vi "Check Workflow.vi"(9 "Part In":map{string, i64}(c390), 10 "Current  Workflow":string, 11 "Workflow Map":map{string, string[]}(c390)) -> (3 "Accepted?":bool)   [LabVIEW 2021]
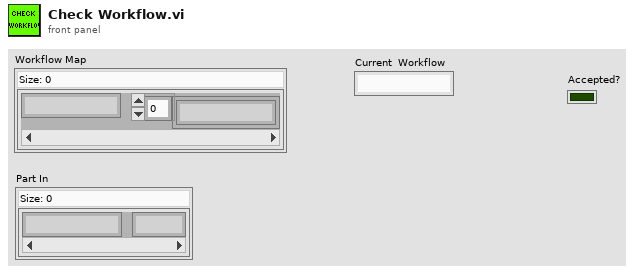
[diagram p1: front panel]
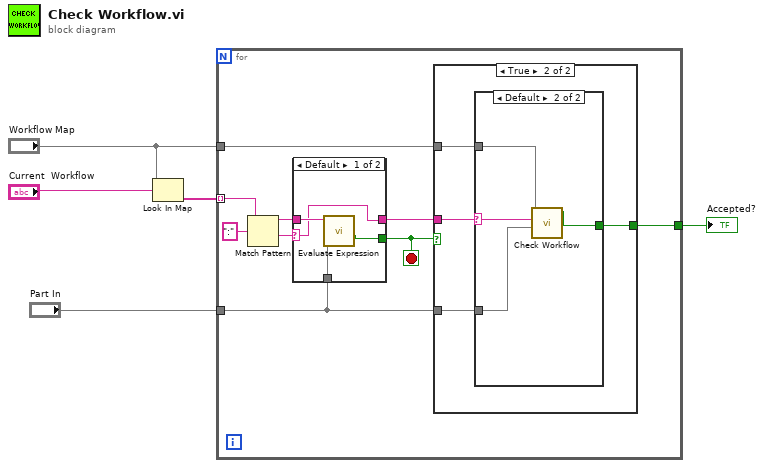
[diagram p0: block diagram]
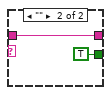
[diagram p2: hidden frame]
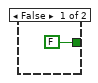
[diagram p3: hidden frame]
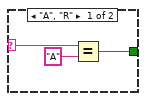
[diagram p4: hidden frame]
diagram:
  n1 = Look In Map(map="Workflow Map", key="Current  Workflow") -> (value=w4:string[])  [unwired: 1 in, 1 out]
  n2 = for {
    tunnel: w4 -> [w14] mode=indexing
    tunnel: "Workflow Map" -> [w8]
    tunnel: "Part In" -> [w6]
    tunnel: [w7] -> w1
    stop <- w9 stop-if-true
    n3 = Match Pattern(string=w14, regular expression=":") -> (before substring=w11:string, after substring=w12:string)  [unwired: 1 in, 2 out]
    n4 = case shown="Default" w12 {
      selector: w12 -> [w15 _]
      tunnel: [w16 TRUE] -> w9
      tunnel: w11 -> [w18 w19]
      tunnel: [w15 w19] -> w10
      tunnel: w6 -> [w17 _]
      frame Default {
        n5 = call "Evaluate Expression.vi"("Part In"=w17, "Expression"=w18) -> ("Pass/Fail"=w16:bool)  [unwired: 9 in]
      }
      frame "" {
      }
    }
    n6 = case shown="True" w9 {
      tunnel: w10 -> [_ w25]
      tunnel: w8 -> [_ w24]
      tunnel: w6 -> [_ w23]
      tunnel: [FALSE w22] -> w7
      frame False {
      }
      frame True {
        n7 = case shown="Default" w25 {
          selector: w25 -> [w28 w30]
          tunnel: w24 -> [_ w32]
          tunnel: w23 -> [_ w31]
          tunnel: [w26 w29] -> w22
          frame "A", "R" {
            n8 = Equal?(x=w28, y="A") -> (x = y?=w26:bool)
          }
          frame Default {
            n9 = call "Check Workflow.vi"("Part In"=w31, "Current  Workflow"=w30, "Workflow Map"=w32) -> ("Accepted?"=w29:bool)  [unwired: 8 in]
          }
        }
      }
    }
  }
  "Accepted?" <- w1
